vi "5x Parameter Regler lesen.vi"(8 "Fehler (Eingang, kein Fehler)":errorcluster, 11 "Dateipfad im Ordner des Haupt-VIs":path) -> (0 "Fehler (Ausgang)":errorcluster, 3 "Parameter Regler":T1)   [LabVIEW 2015, in "allgemeine Sub-VIs.lvlib"]
uses:
  allgemeine Sub-VIs.lvlib
  cRIO/PC/Parameter Druckregler.ctl
  cRIO/PC/Kommunikation mit cRIO.lvlib
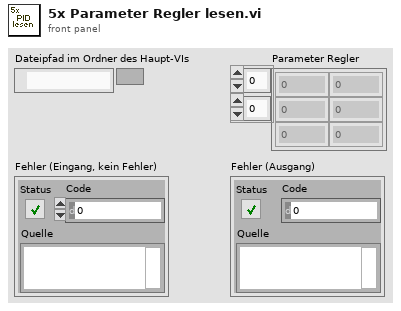
[diagram p1: front panel]
types:
  T1 = typedef "Kommunikation mit cRIO.lvlib/Parameter Druckregler.ctl" = sgl[][]
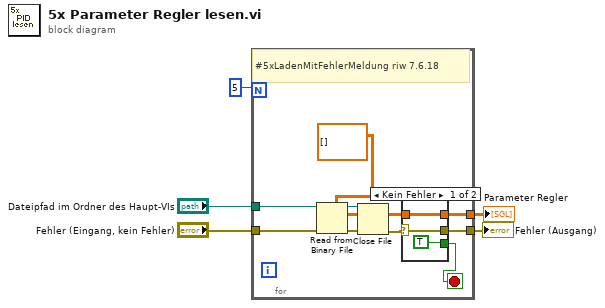
[diagram p0: block diagram]
diagram:
  n1 = for {
    N: 5 -> [_]
    tunnel: [w11] -> w1
    tunnel: "Dateipfad im Ordner des Haupt-VIs" -> [w14]
    tunnel: "Fehler (Eingang, kein Fehler)" -> [w15]
    tunnel: [w13] -> w5
    stop <- w10 stop-if-true
    # "#5xLadenMitFehlerMeldung riw 7.6.18"
    n2 = Read from Binary File(5:T1 [] ("Parameter Regler"), 8:w15, 11:w14) -> (0:w8:errorcluster, 2:w12:T1, 3:w9:refnum<file>)  [unwired: 1 in, 3 out]
    n3 = Close File(refnum=w9, error in=w8) -> (error out=w7:errorcluster)  [unwired: 1 out]
    n4 = case shown="Kein Fehler" w7 {
      selector: w7 -> [w18 w20]
      tunnel: [w18 w20] -> w13
      tunnel: w12 -> [w17 w19]
      tunnel: [w17 w19] -> w11
      tunnel: [TRUE _] -> w10
      frame No Error {
      }
      frame Error {
      }
    }
  }
  "Fehler (Ausgang)" <- w5
  "Parameter Regler" <- w1
